vi "SingleAcquisitionDisplayImageData.vi"() -> ()   [LabVIEW 2018]
uses:
  C:/Users/Public/Documents/Photometrics/PMQI-LabViewSamples/Examples/Dependencies/PVCamNET.dll
  Public/Documents/Photometrics/PMQI-LabViewSamples/Examples/Dependencies/PVCamNET.dll
panel:
  out "Min":dbl
  out "Max":dbl
  out "RawImageData":i32[](array[numeric])
  out "Waveform Graph":i32[](graph)
  out "Boolean 2":bool
  out "Boolean":bool
  in  "?":bool
  in  "?":bool
  in  "Exposure time":dbl=30.0
  in  "?":bool
  # "SingleAcquisitionDisplayImageData.vi\n\nDescription:\nThis sample code lets the user access the image data from the buffer.\n\nSteps to run:\n1. Click \"Run\"\n2. Enter exposure time\n3. Click \"START\"\n4. Click \"DISPLAY\"\n5. Click \"CLOSE\""
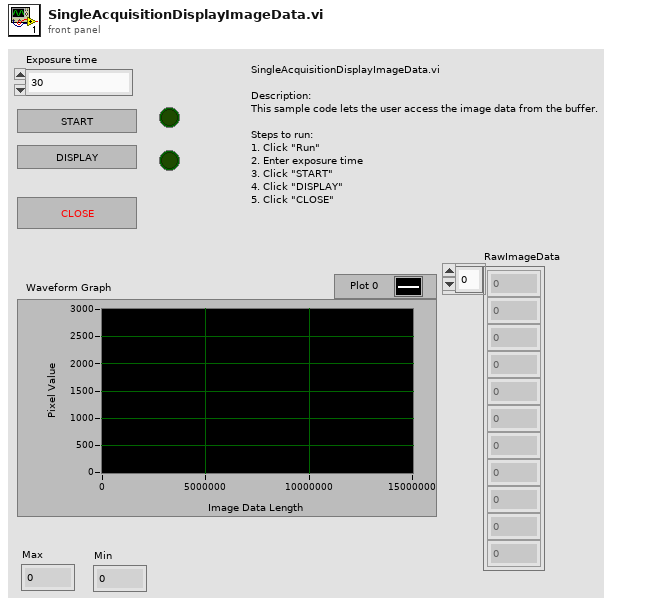
[diagram p1: front panel]
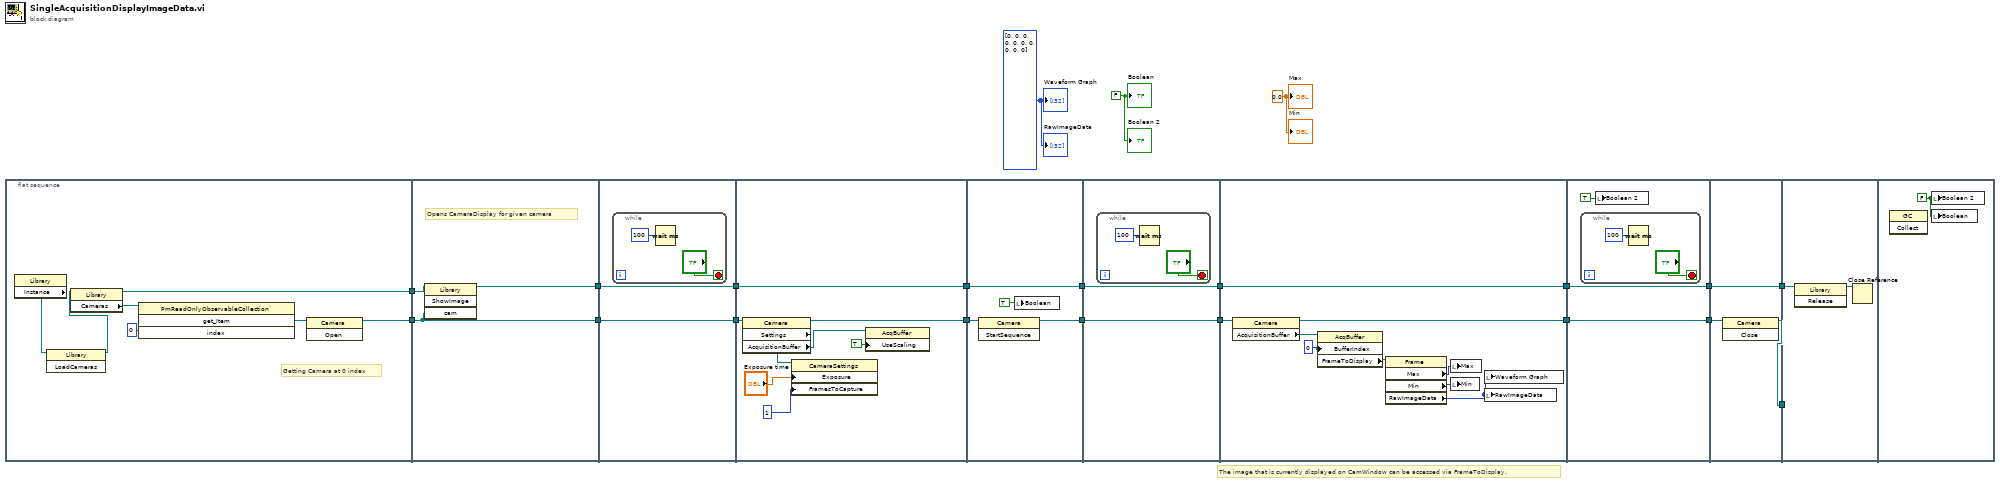
[diagram p0: block diagram]
diagram:
  w1 = 0.0 ("Max")
  w2 = i32[] [0, 0, 0, 0, 0, 0, 0, 0, 0, 0] ("RawImageData")
  w5 = FALSE ("Boolean")
  # "The image that is currently displayed on CamWindow can be accessed via FrameToDisplay."
  n1 = flat-sequence {
    tunnel: [w24] -> w21
    tunnel: [w25] -> w20
    tunnel: w21 -> [w31]
    tunnel: w20 -> [w30]
    tunnel: [w30] -> w19
    tunnel: [w29] -> w18
    tunnel: w19 -> [w33]
    tunnel: [w33] -> w16
    tunnel: w18 -> [w32]
    tunnel: [w32] -> w17
    tunnel: [w43] -> w15
    tunnel: [w42] -> w14
    tunnel: w17 -> [w42]
    tunnel: w16 -> [w41]
    tunnel: w15 -> [w46]
    tunnel: [w45] -> w9
    tunnel: [w47] -> w7
    tunnel: w14 -> [w47]
    tunnel: w9 -> [w49]
    tunnel: [w49] -> w8
    tunnel: w7 -> [w48]
    tunnel: [w48] -> w6
    tunnel: w8 -> [w59]
    tunnel: [w56] -> w4
    tunnel: w6 -> [w60]
    tunnel: [w60] -> w3
    tunnel: w4 -> [w63]
    tunnel: [w63] -> w11
    tunnel: w3 -> [w62]
    tunnel: [w62] -> w10
    tunnel: w11 -> [w68]
    tunnel: w10 -> [w66]
    tunnel: [w67] -> w13
    tunnel: [w66] -> w12
    tunnel: w13 -> [_]
    tunnel: w12 -> [w70]
    frame #0 {
      # "Getting Camera at 0 index"
      n2 = property class="Library"() -> ("Instance"=w23:refnum<k24>)  [unwired: 2 in, 2 out]
      n3 = invoke class="Library" method="LoadCameras"(reference=w23) -> (reference out=w22:refnum<k24>)  [unwired: 2 in, 2 out]
      n4 = property class="Library"(reference=w22) -> (reference out=w24:refnum<k24>, "Cameras"=w28:refnum<k24>)  [unwired: 1 in, 1 out]
      n5 = invoke class="PmReadOnlyObservableCollection`" method="get_Item"(reference=w28, "index"=0) -> ("get_Item"=w26:refnum<k24>)  [unwired: 2 in, 3 out]
      n6 = invoke class="Camera" method="Open"(reference=w26) -> (reference out=w25:refnum<k24>)  [unwired: 2 in, 2 out]
    }
    frame #1 {
      # "Opens CameraDisplay for given camera"
      n7 = invoke class="Library" method="ShowImage"(reference=w31, "cam"=w30) -> (reference out=w29:refnum<k24>)  [unwired: 2 in, 3 out]
    }
    frame #2 {
      n8 = while {
        stop <- "?" stop-if-true
        n9 = Wait (ms)(milliseconds to wait=u32 100) -> ()  [unwired: 1 out]
      }
    }
    frame #3 {
      n10 = property class="Camera"(reference=w41) -> (reference out=w43:refnum<k24>, "Settings"=w39:refnum<k24>, "AcquisitionBuffer"=w37:refnum<k24>)  [unwired: 1 in, 1 out]
      n11 = property class="CameraSettings"(reference=w39, "Exposure"="Exposure time", "FramesToCapture"=u16 1) -> ()  [unwired: 1 in, 2 out]
      n12 = property class="AcqBuffer"(reference=w37, "UseScaling"=TRUE) -> ()  [unwired: 1 in, 2 out]
    }
    frame #4 {
      n13 = invoke class="Camera" method="StartSequence"(reference=w46) -> (reference out=w45:refnum<k24>)  [unwired: 2 in, 2 out]
      n14 = local write "Boolean"(TRUE ("Boolean")) -> ()
    }
    frame #5 {
      n15 = while {
        stop <- "?" stop-if-true
        n16 = Wait (ms)(milliseconds to wait=u32 100) -> ()  [unwired: 1 out]
      }
    }
    frame #6 {
      n17 = property class="Camera"(reference=w59) -> (reference out=w56:refnum<k24>, "AcquisitionBuffer"=w58:refnum<k24>)  [unwired: 1 in, 1 out]
      n18 = property class="AcqBuffer"(reference=w58, "BufferIndex"=0) -> ("FrameToDisplay"=w53:refnum<k24>)  [unwired: 1 in, 2 out]
      n19 = property class="Frame"(reference=w53) -> ("Max"=w55:u32, "Min"=w54:u32, "RawImageData"=w52:i16[])  [unwired: 1 in, 2 out]
      n20 = local write "Max"(w55) -> ()
      n21 = local write "Min"(w54) -> ()
      n22 = local write "Waveform Graph"(w52) -> ()
      n23 = local write "RawImageData"(w52) -> ()
    }
    frame #7 {
      n24 = while {
        stop <- "?" stop-if-true
        n25 = Wait (ms)(milliseconds to wait=u32 100) -> ()  [unwired: 1 out]
      }
      n26 = local write "Boolean 2"(TRUE ("Boolean 2")) -> ()
    }
    frame #8 {
      n27 = invoke class="Camera" method="Close"(reference=w68) -> (reference out=w67:refnum<k24>)  [unwired: 2 in, 2 out]
    }
    frame #9 {
      n28 = invoke class="Library" method="Release"(reference=w70) -> (reference out=w69:refnum<k24>)  [unwired: 2 in, 2 out]
      n29 = Close Reference(reference=w69) -> ()  [unwired: 1 in, 1 out]
    }
    frame #10 {
      w71 = FALSE ("Boolean 2")
      n30 = invoke class="GC" method="Collect"() -> ()  [unwired: 3 in, 3 out]
      n31 = local write "Boolean 2"(w71) -> ()
      n32 = local write "Boolean"(w71) -> ()
    }
  }
  "Boolean" <- w5
  "Boolean 2" <- w5
  "RawImageData" <- w2
  "Waveform Graph" <- w2
  "Max" <- w1
  "Min" <- w1
